vi "lab2(dll;works).vi"() -> ()   [LabVIEW 2016]
uses:
  lab2RbgDll.dll
panel:
  out "2D Picture":picture
  in  "SwapGB":bool
  in  "SwapRB":bool
  in  "SwapRG":bool
  in  "Original":bool
  in  "ImagePath":path
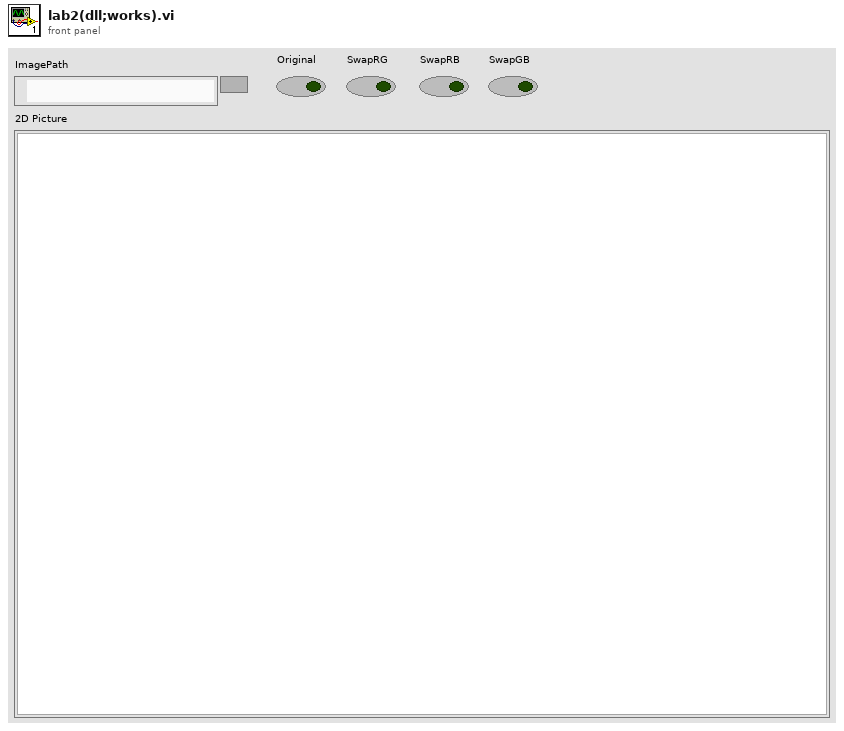
[diagram p1: front panel]
types:
  T1 = typedef "imagedata.ctl" = cluster{"image type":i32, "image depth":i32, "image":u8[], "mask":u8[], "colors":u32[], "Rectangle":cluster{"left":i16, "top":i16, "right":i16, "bottom":i16}}
  T2 = cluster{"left":i16, "top":i16, "right":i16, "bottom":i16}
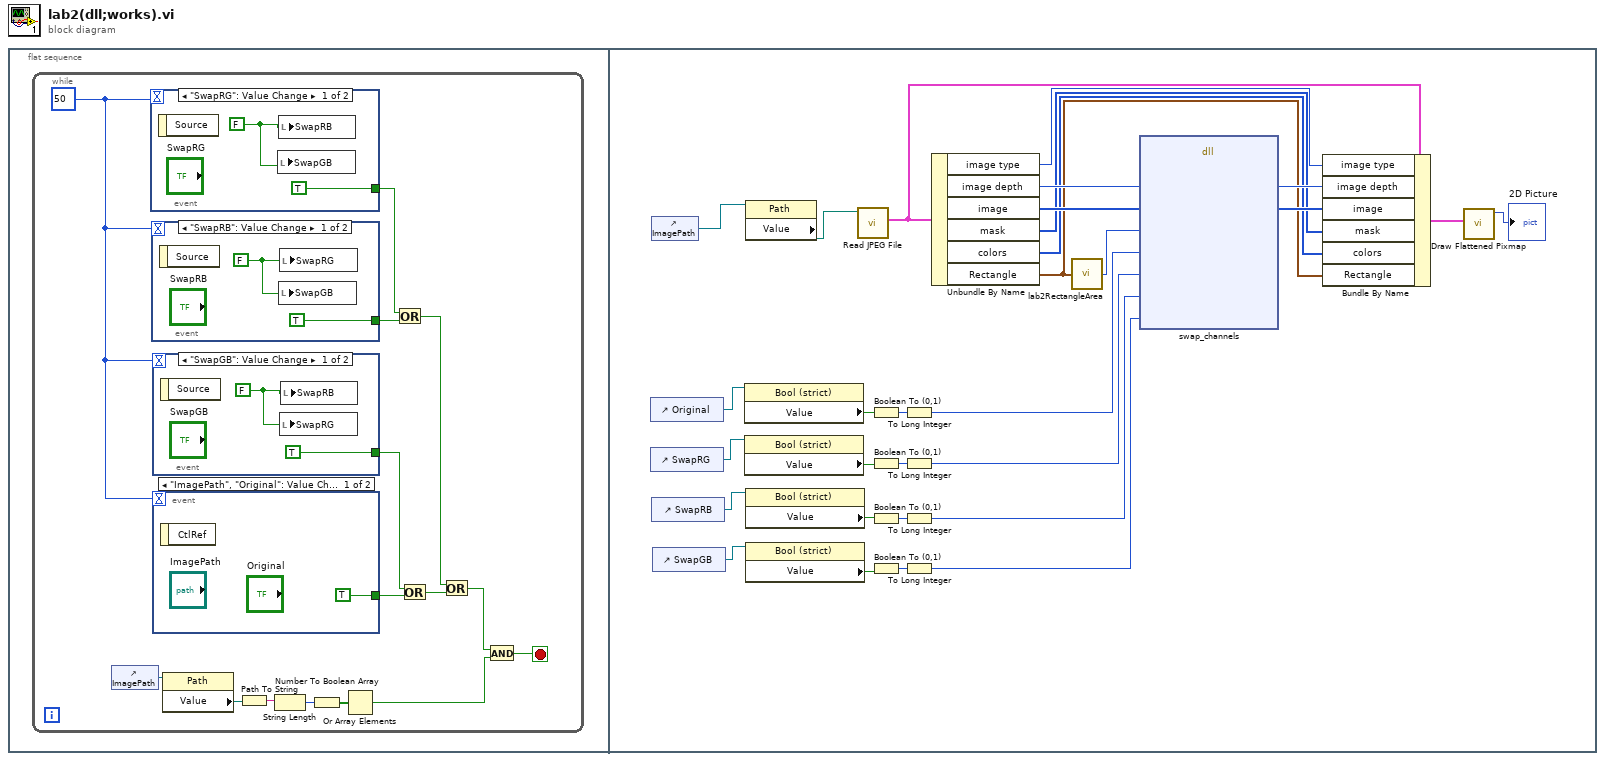
[diagram p0: block diagram]
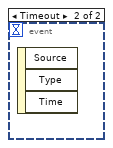
[diagram p2: hidden frame]
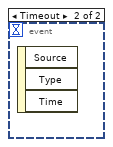
[diagram p3: hidden frame]
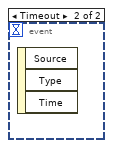
[diagram p4: hidden frame]
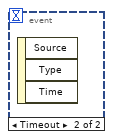
[diagram p5: hidden frame]
diagram:
  n1 = flat-sequence {
    frame #0 {
      n2 = while {
        stop <- w3 stop-if-true
        w11 = 50
        n3 = control-ref of="ImagePath"() -> (w15:refnum<vi>)
        n4 = event shown="[0] \"SwapRG\": Value Change" {
          selector: _ -> [_ _]
          dyn-events: _ -> [_ _]
          timeout: w11 -> [_ _]
          tunnel: [TRUE _] -> w5
          event "SwapRG": Value Change {
            w21 = FALSE
            n5 = event-data() -> ()  [unwired: 1 in, 1 out]
            n6 = local write "SwapGB"(w21) -> ()
            n7 = local write "SwapRB"(w21) -> ()
          }
          event Timeout {
            n8 = event-data() -> ()  [unwired: 1 in, 3 out]
          }
        }
        n9 = event shown="[0] \"SwapRB\": Value Change" {
          selector: _ -> [_ _]
          dyn-events: _ -> [_ _]
          timeout: w11 -> [_ _]
          tunnel: [TRUE _] -> w8
          event "SwapRB": Value Change {
            w19 = FALSE
            n10 = event-data() -> ()  [unwired: 1 in, 1 out]
            n11 = local write "SwapGB"(w19) -> ()
            n12 = local write "SwapRG"(w19) -> ()
          }
          event Timeout {
            n13 = event-data() -> ()  [unwired: 1 in, 3 out]
          }
        }
        n14 = event shown="[0] \"SwapGB\": Value Change" {
          selector: _ -> [_ _]
          dyn-events: _ -> [_ _]
          timeout: w11 -> [_ _]
          tunnel: [TRUE _] -> w4
          event "SwapGB": Value Change {
            w17 = FALSE
            n15 = event-data() -> ()  [unwired: 1 in, 1 out]
            n16 = local write "SwapRG"(w17) -> ()
            n17 = local write "SwapRB"(w17) -> ()
          }
          event Timeout {
            n18 = event-data() -> ()  [unwired: 1 in, 3 out]
          }
        }
        n19 = event shown="[0] \"ImagePath\", \"Original\": Value Change" {
          selector: _ -> [_ _]
          dyn-events: _ -> [_ _]
          timeout: w11 -> [_ _]
          tunnel: [TRUE _] -> w9
          event "ImagePath", "Original": Value Change {
            n20 = event-data() -> ()  [unwired: 1 in, 1 out]
          }
          event Timeout {
            n21 = event-data() -> ()  [unwired: 1 in, 3 out]
          }
        }
        n22 = property class="Path"(reference=w15) -> ("Value"=w14:path)  [unwired: 1 in, 2 out]
        n23 = Path To String(path=w14) -> (string=w13:string)
        n24 = String Length(string=w13) -> (length=w10:i32)
        n25 = Number To Boolean Array(number=w10) -> (Boolean array=w12:bool[])
        n26 = Or Array Elements(Boolean array=w12) -> (logical OR=w1:bool)
        n27 = Or(x=w5, y=w8) -> (x .or. y?=w6:bool)
        n28 = Or(x=w4, y=w9) -> (x .or. y?=w7:bool)
        n29 = Or(x=w6, y=w7) -> (x .or. y?=w2:bool)
        n30 = And(x=w2, y=w1) -> (x .and. y?=w3:bool)
      }
    }
    frame #1 {
      n31 = control-ref of="Original"() -> (w50:refnum<vi>)
      n32 = control-ref of="SwapRG"() -> (w49:refnum<vi>)
      n33 = control-ref of="ImagePath"() -> (w51:refnum<vi>)
      n34 = control-ref of="SwapRB"() -> (w48:refnum<vi>)
      n35 = control-ref of="SwapGB"() -> (w47:refnum<vi>)
      n36 = property class="Bool (strict)"(reference=w50) -> ("Value"=w42:bool)  [unwired: 1 in, 2 out]
      n37 = property class="Bool (strict)"(reference=w49) -> ("Value"=w41:bool)  [unwired: 1 in, 2 out]
      n38 = property class="Path"(reference=w51) -> ("Value"=w43:path)  [unwired: 1 in, 2 out]
      n39 = property class="Bool (strict)"(reference=w48) -> ("Value"=w39:bool)  [unwired: 1 in, 2 out]
      n40 = property class="Bool (strict)"(reference=w47) -> ("Value"=w40:bool)  [unwired: 1 in, 2 out]
      n41 = call <vilib>:"Read JPEG File.vi"("path to JPEG file"=w43) -> ("image data"=w38:T1)  [unwired: 8 in, 2 out]
      n42 = Boolean To (0,1)(Boolean=w42) -> (0, 1=w30:i16)
      n43 = Boolean To (0,1)(Boolean=w41) -> (0, 1=w28:i16)
      n44 = Boolean To (0,1)(Boolean=w39) -> (0, 1=w27:i16)
      n45 = Boolean To (0,1)(Boolean=w40) -> (0, 1=w26:i16)
      n46 = To Long Integer(number=w30) -> (32bit integer=w29:i32)
      n47 = To Long Integer(number=w28) -> (32bit integer=w25:i32)
      n48 = To Long Integer(number=w27) -> (32bit integer=w24:i32)
      n49 = To Long Integer(number=w26) -> (32bit integer=w23:i32)
      n50 = Unbundle By Name(w38) -> ("image type"=w36:i32, "image depth"=w46:i32, "image"=w45:u8[], "mask"=w33:u8[], "colors"=w32:u32[], "Rectangle"=w31:T2)
      n51 = call "lab2RectangleArea.vi"("Rectangle"=w31) -> ("Area"=w44:u32)
      n52 = dll-call lib="PTH2Mabs DDropboxTETSмагалабыapgslab2antonlab2RbgDll.dll" fn="swap_channels"("image_depth"=w46, "image"=w45, "image_size"=w44, "bypass"=w29, "swap_rg"=w25, "swap_rb"=w24, "swap_gb"=w23) -> ("image_depth"=w35:i32, "image"=w34:u8[])  [unwired: 9 in, 2 out]
      n53 = Bundle By Name(cluster=w38, "image type"=w36, "image depth"=w35, "image"=w34, "mask"=w33, "colors"=w32, "Rectangle"=w31) -> (w37:T1)
      n54 = call <vilib>:"Draw Flattened Pixmap.vi"("image data"=w37) -> ("new picture"=→"2D Picture":picture)  [unwired: 8 in]
    }
  }
